vi "GetControllerName.vi"(8 "error in (no error)":errorcluster, 11 "controller in":refnum<k24>) -> (0 "error out":errorcluster, 2 "ControllerName":string, 3 "controller out":refnum<k24>)   [LabVIEW 2019]
uses:
  C:/Users/patrick/Documents/GitHub/Aerotech-Delay-Line/lvsrc/Aerotech-Ensemble-LabVIEW/2010-5.6/Bin/Aerotech.Ensemble.dll
  Bin/Aerotech.Ensemble.dll
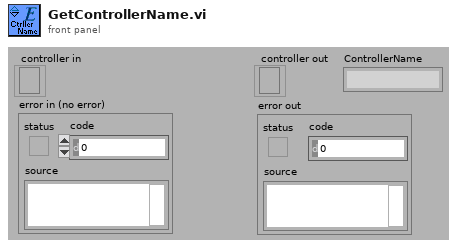
[diagram p1: front panel]
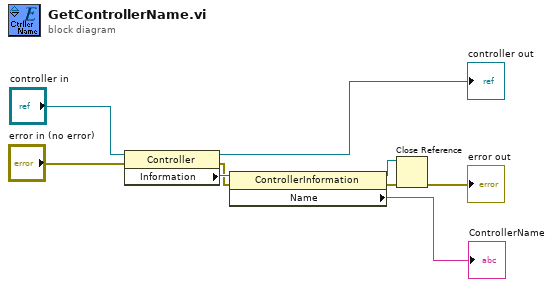
[diagram p0: block diagram]
diagram:
  n1 = property class="Controller"(reference="controller in", error in="error in (no error)") -> (reference out=→"controller out":refnum<k24>, error out=w8:errorcluster, "Information"=w9:refnum<k24>)
  n2 = property class="ControllerInformation"(reference=w9, error in=w8) -> (reference out=w6:refnum<k24>, error out=w7:errorcluster, "Name"=→"ControllerName":string)
  n3 = Close Reference(reference=w6, error in (no error)=w7) -> (error out=→"error out":errorcluster)
